vi "DB - [CMS].[Execute].[ActiveProcess].vi"(0 "connection reference":T3, 2 "Application":string, 3 "String ([RawDataFile] Filestream)":string, 4 "[PlantId],[SystemId]":cluster{"[PlantId]":string, "[SystemId]":string}, 5 "error in (no error)":errorcluster, 6 "DB Connection":T4={"Open"=TRUE, "Close"=TRUE}, 7 "Filestream Position (0/<int>/NULL)":string, 8 "DB - CMS Execute ActiveProcess":T2, 9 "Skip TimeStamps":bool, 10 "[Execute].[ActiveProcess]\n2014-10-14 14:58":T1[](array[typedef]), 12 "<Data>":string[](array[string])) -> (14 "connection reference":T3, 15 "data":string[](array[string]), 17 "String ([RawDataFile] Filestream)":string, 19 "SUMMARY":errorcluster)   [LabVIEW 2013]
uses:
  <vilib>/addons/database/Connection.llb/Conn ObjectReference.ctl
  Controls/DB - OpenClose.ctl
  Controls/DB - CMS Execute Active Process.ctl
  Controls/DB - [Execute].[ActiveProcess] Enum.ctl
  Controls/Global CMS.vi
  Controls/Global SRTRS.vi
  <vilib>/addons/database/Connection.llb/DB Tools Open Connec (String).vi
  <vilib>/addons/database/Connection.llb/Conn Execute.vi
  <vilib>/addons/database/Recordset.llb/Rec Destroy - Connection.vi
  <vilib>/addons/database/Recordset.llb/Rec Fetch Recordset Data (R).vi
  <vilib>/addons/database/NI_Database_API.lvlib
panel:
  out "Filestream":string
  out "Close":errorcluster
  out "SQL Statement":string
  in  "DB.Schema.Table \n(NA)":string
  in  "CMS.Execute.ActiveProcess":string="CMS.Execute.ActiveProcess"
  out "CMS Connection Information":T5={"Connection "="SQL Server 32bit HPEnvy", "Username"="admin", "Password"="admin123"}
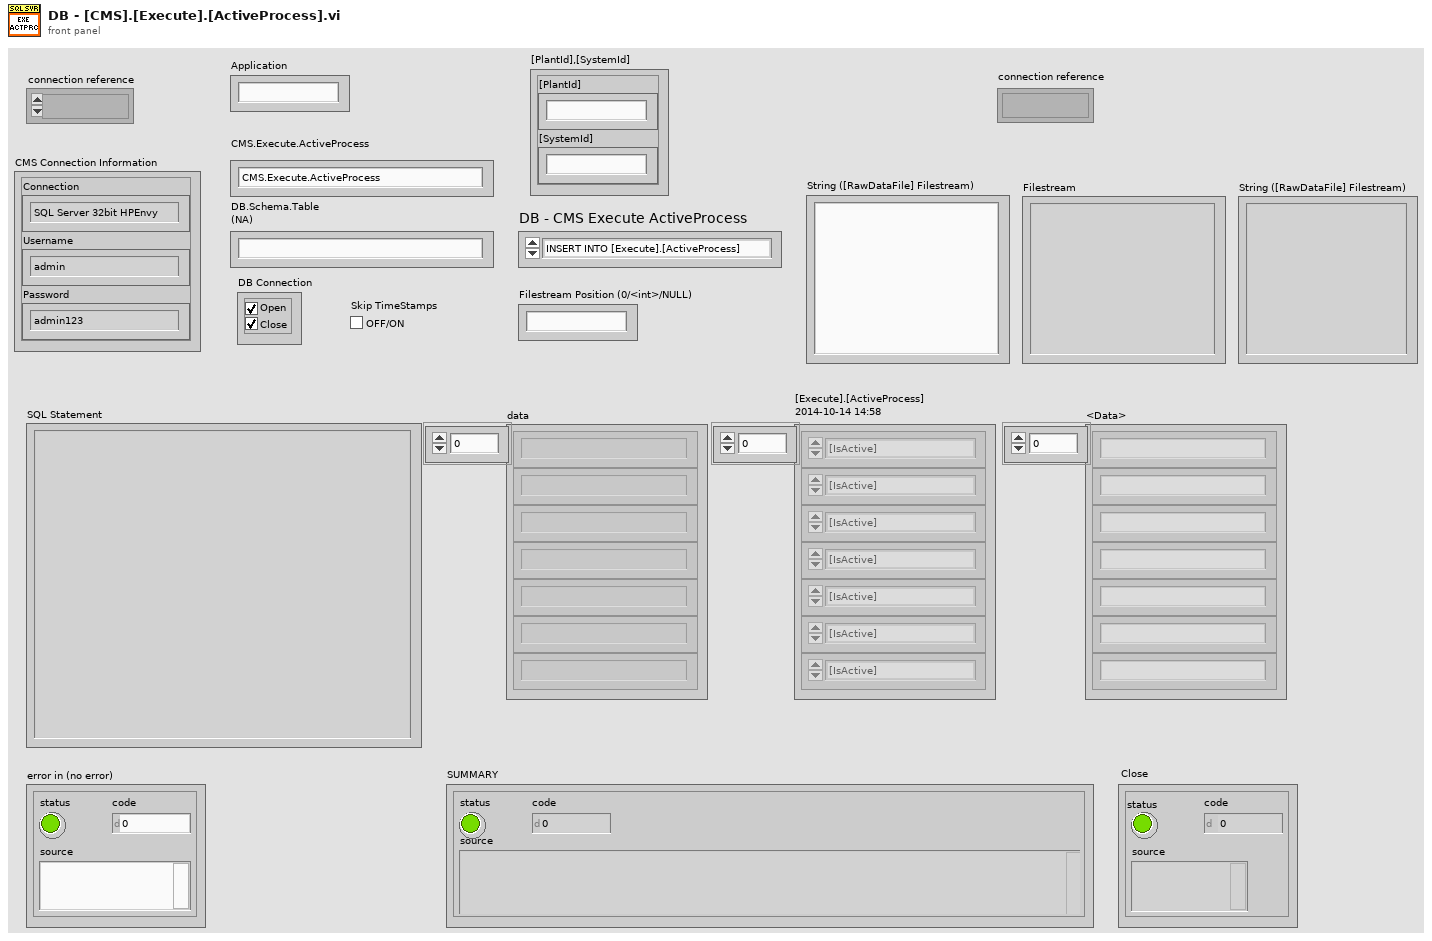
[diagram p1: front panel]
types:
  T1 = typedef "DB - [Execute].[ActiveProcess] Enum.ctl" = enum16{"[IsActive]", "[TransactionNo]", "[TransactionRunNo]", "[SequenceStatus]", "[StartRecordTime]", "[EndRecordTime]", "[StartHoldTime]", "[EndHoldTime]", "[Message1]", "[Message2]", "[HoldTimeRemaining]", "[HoldTimePercentage]", "[HoldProgressColor]", "[OrderNumbers]", "[CurrentTemp]", "[UnitOfTemperature]", "[IsAppClientLive]", "[RawDataFile]", "[RecordedMinutes]", "[FurnaceControlStatus]", "[FurnaceControlColor]", "[ControllerStatus]", "[ControllerColor]", "[IsControllerOnline]", "[ProcessColor]", "[OverallColor]", "[LastUpdatedOn]", "[LastUpdatedCmsTime]", "[Inactive]"}
  T2 = typedef "DB - CMS Execute Active Process.ctl" = enum16{"INSERT INTO [Execute].[ActiveProcess]", "UPDATE [Execute].[ActiveProcess]", "SELECT [Execute].[ActiveProcess]", "UPDATE FILESTREAM", "SELECT FILESTREAM", "Check [IsActive]"}
  T3 = typedef "NI_Database_API.lvlib/Conn ObjectReference.ctl" = refnum<k1>
  T4 = typedef "DB - OpenClose.ctl" = cluster{"Open":bool, "Close":bool}
  T5 = cluster{"Connection ":string, "Username":string, "Password":string}
  T6 = typedef "Enum - InteractiveMode-SubVIMode.ctl" = enum16{"Interactive", "subVI Mode"}
  T7 = typedef "Connection Information Cluster.ctl" = cluster{"Connection ":string, "Username":string, "Password":string}
  T8 = typedef "DB - DB.Schema.Table.ctl" = cluster{"DB":string, "Schema":string, "Table":string}
  T9 = typedef "NI_Database_API.lvlib/Rec ObjectReference.ctl" = refnum<k1>
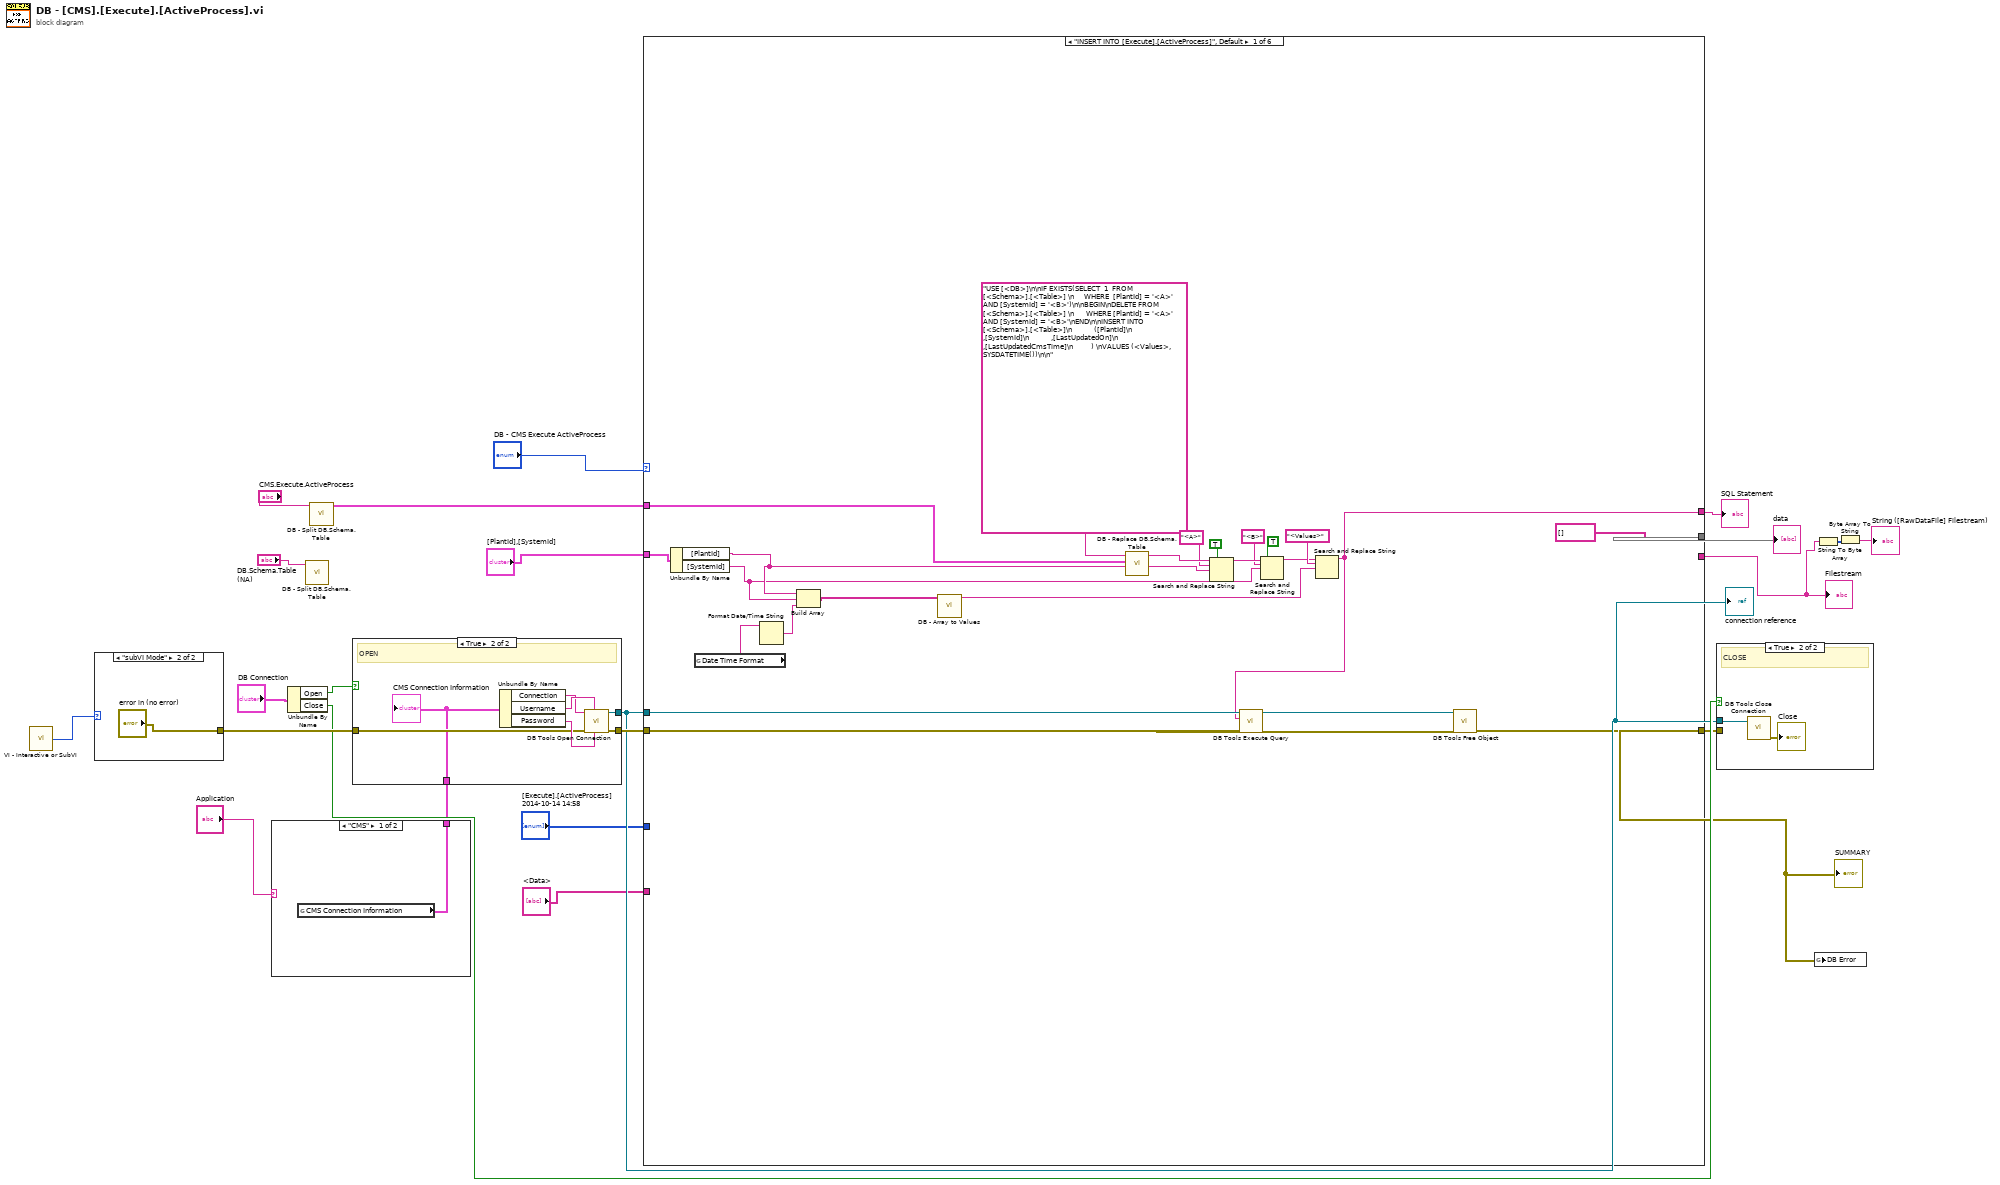
[diagram p0: block diagram]
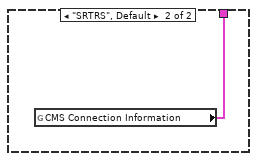
[diagram p2: hidden frame]
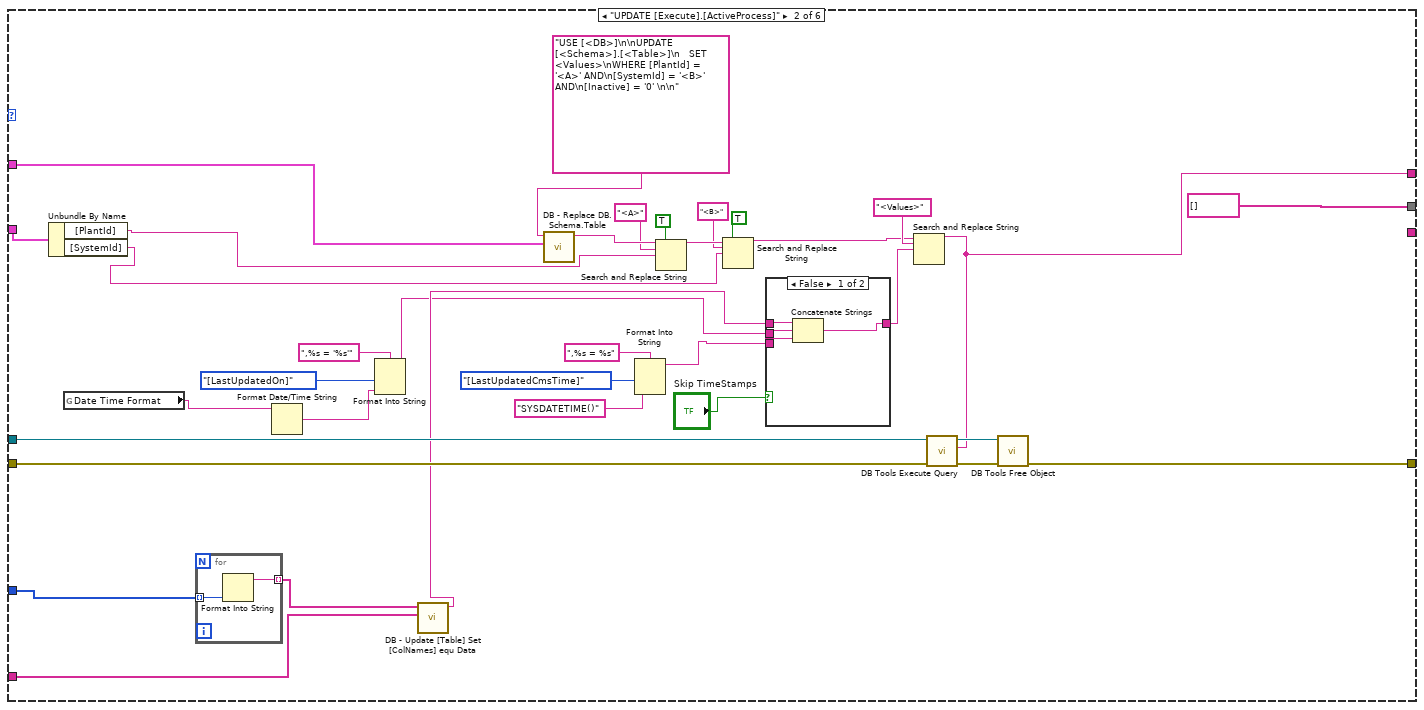
[diagram p3: hidden frame]
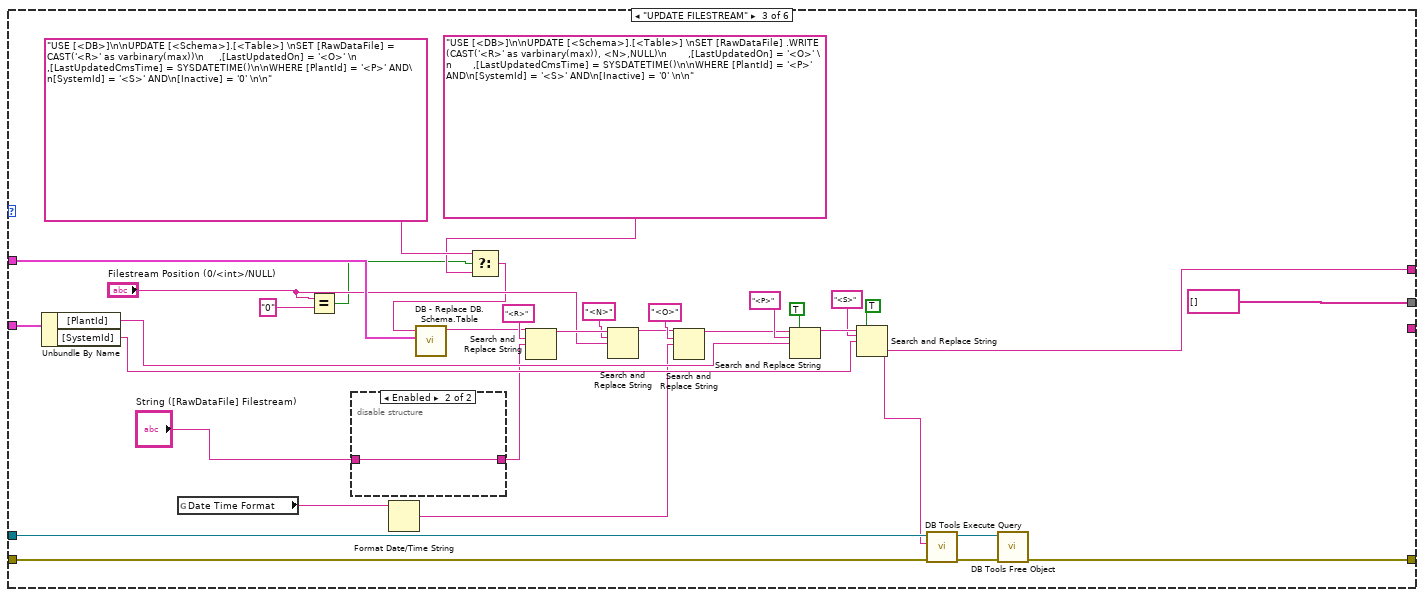
[diagram p5: hidden frame]
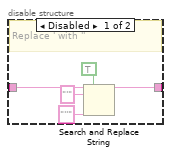
[diagram p6: hidden frame]
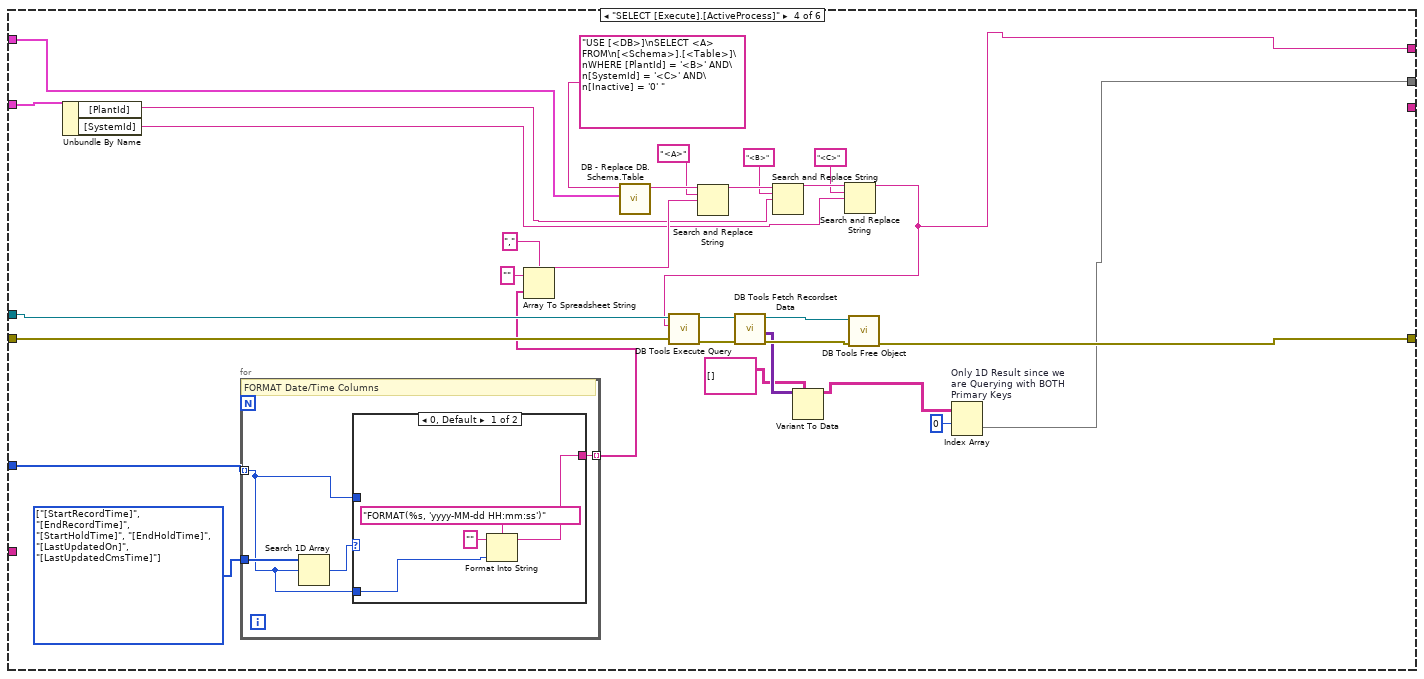
[diagram p7: hidden frame]
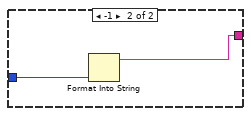
[diagram p8: hidden frame]
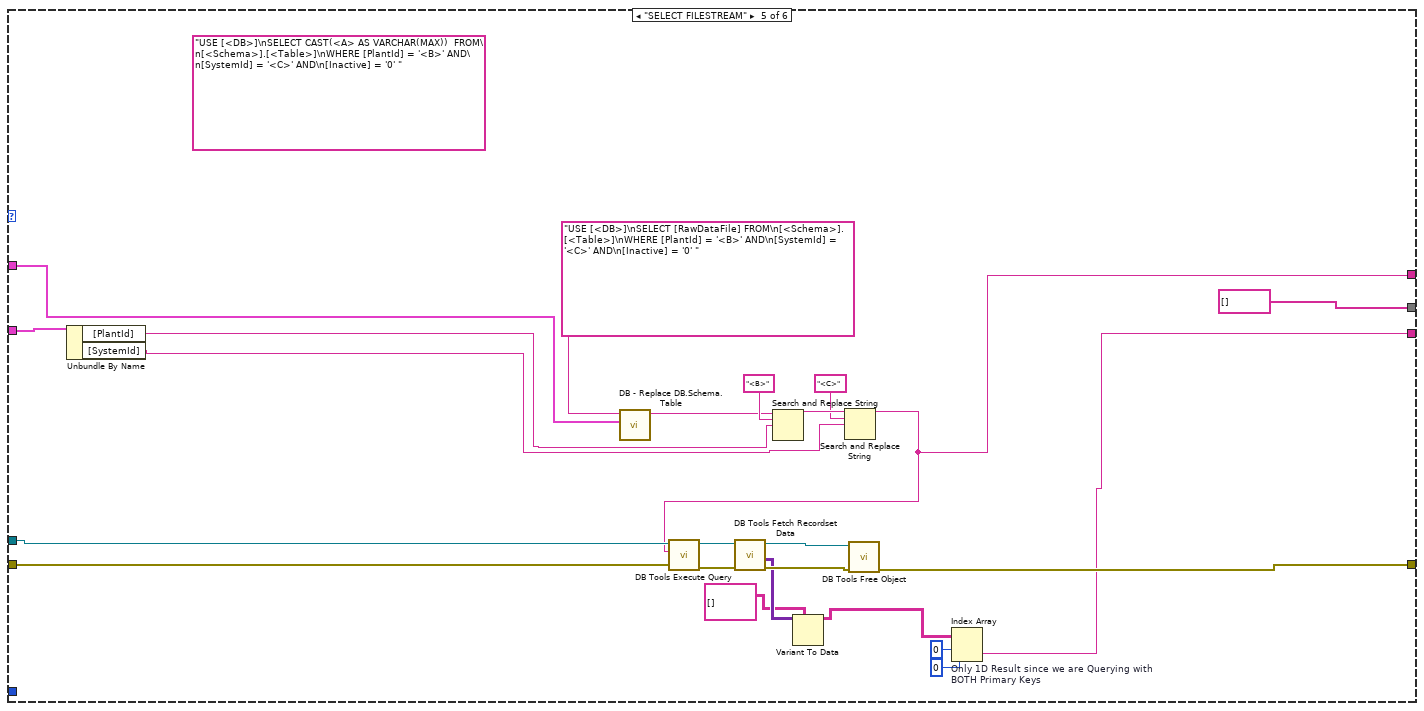
[diagram p9: hidden frame]
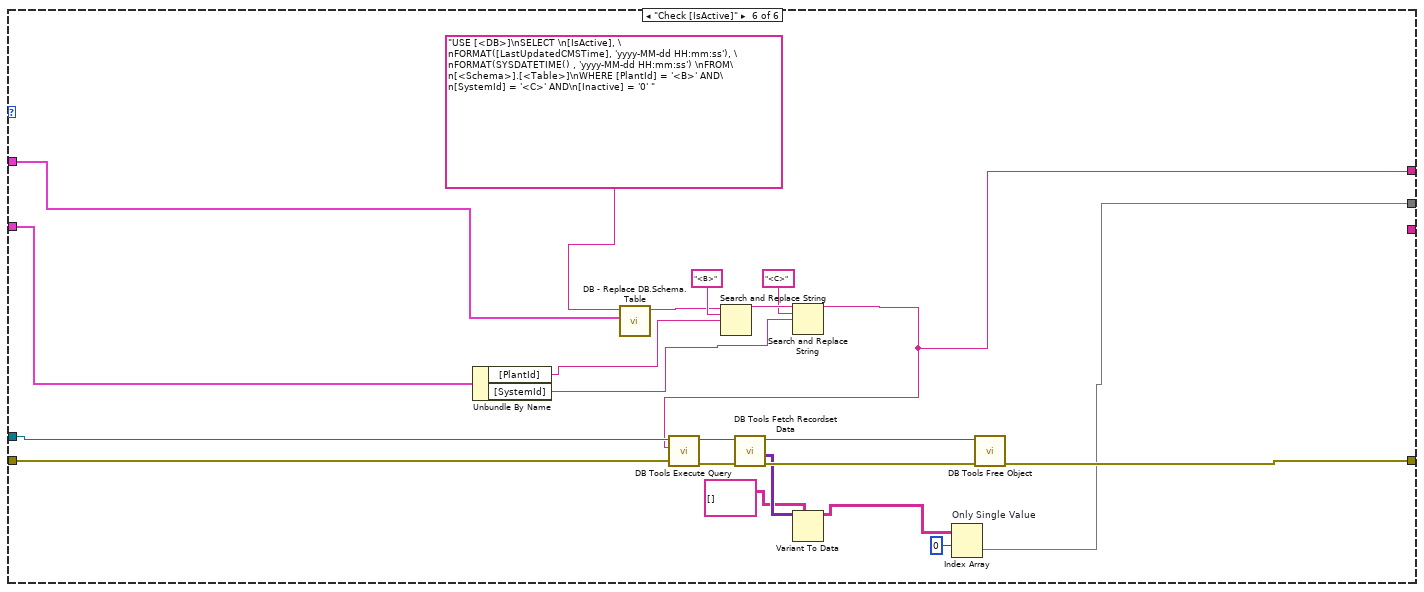
[diagram p10: hidden frame]
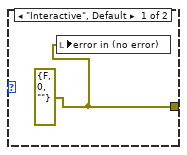
[diagram p12: hidden frame]
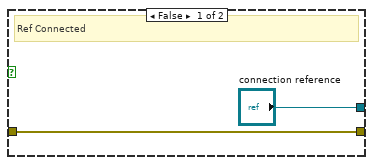
[diagram p13: hidden frame]
diagram:
  n1 = call "VI - Interactive or SubVI.vi"() -> ("Mode"=w20:T6)  [unwired: 5 in]
  n2 = case shown="\"subVI Mode\"" w20 {
    tunnel: [w23 "error in (no error)"] -> w19
    frame "Interactive", Default {
      w23 = errorcluster {"status"=FALSE, "code"=0, "source"=""} ("error in (no error)")
      n3 = local write "error in (no error)"(w23) -> ()
    }
    frame "subVI Mode" {
    }
  }
  n4 = case shown="\"CMS\"" "Application" {
    tunnel: [w25 w26] -> w1
    frame "CMS" {
      n5 = global read "Global CMS.vi" "CMS Connection Information"() -> (w25:T7)
    }
    frame "SRTRS", Default {
      n6 = global read "Global SRTRS.vi" "CMS Connection Information"() -> (w26:T7)
    }
  }
  n7 = Unbundle By Name("DB Connection") -> ("Open"=w21:bool, "Close"=w17:bool)
  n8 = call "DB - Split DB.Schema.Table.vi"("DB.Schema.Table"="DB.Schema.Table \n(NA)") -> ()  [unwired: 10 in, 1 out]
  n9 = call "DB - Split DB.Schema.Table.vi"("DB.Schema.Table"="CMS.Execute.ActiveProcess") -> ("DB.Schema.Table"=w14:T8)  [unwired: 10 in]
  n10 = case shown="True" w21 {
    tunnel: ["connection reference" w32] -> w10
    tunnel: w19 -> [w27 w31]
    tunnel: [w27 w30] -> w18
    tunnel: w1 -> [_ w29]
    frame False {
      # "Ref Connected"
    }
    frame True {
      # "OPEN"
      n11 = Unbundle By Name(w29) -> ("Connection"=w34:string, "Username"=w35:string, "Password"=w33:string)
      n12 = call-poly <vilib>:"DB Tools Open Connection.vi"("password"=w33, "userID"=w35, "error in (no error)"=w31, "connection information"=w34) -> ("error out"=w30:errorcluster, "connection reference"=w32:T3)  [unwired: 4 in]
      "CMS Connection Information" <- w29
    }
  }
  "connection reference" <- w10
  n13 = case shown="\"INSERT INTO [Execute].[ActiveProcess]\", Default" "DB - CMS Execute ActiveProcess" {
    tunnel: w10 -> [w59 w83 w127 w152 w192 w218]
    tunnel: w18 -> [w58 w84 w128 w151 w191 w217]
    tunnel: w14 -> [w57 w86 w129 w147 w188 w215]
    tunnel: [w54 w80 w124 w150 w190 w216] -> w13
    tunnel: [w46 w79 w120 w148 w189 w208] -> w12
    tunnel: "[Execute].[ActiveProcess]\n2014-10-14 14:58" -> [_ w67 _ w143 _ _]
    tunnel: "<Data>" -> [_ w65 _ _ _ _]
    tunnel: [string[] [] string[] [] string[] [] w149 string[] [] w213] -> w7
    tunnel: [_ _ _ _ w185 _] -> w4
    tunnel: "[PlantId],[SystemId]" -> [w38 w74 w119 w146 w184 w207]
    frame "INSERT INTO [Execute].[ActiveProcess]", Default {
      n14 = Unbundle By Name(w38) -> ("[PlantId]"=w37:string, "[SystemId]"=w36:string)
      n15 = global read "Global SRTRS.vi" "Date Time Format"() -> (w40:string)
      n16 = Format Date/Time String(time format string (%c)=w40) -> (date/time string=w39:string)  [unwired: 2 in]
      n17 = Build Array(w37, w36, w39) -> (w41:string[])
      n18 = call "DB - Array to Values.vi"("Array (0xFFFE autodetect)"=w41) -> ("<Values>"=w45:string)  [unwired: 10 in]
      n19 = call "DB - Replace DB.Schema.Table.vi"("DB.Schema.Table"=w57, "string in"="USE [<DB>]\n\nIF EXISTS(SELECT  1  FROM [<Schema>].[<Table>] \n     WHERE  [PlantId] = '<A>'  AND [SystemId] = '<B>')\n\nBEGIN\nDELETE FROM [<Schema>].[<Table>] \n      WHERE [PlantId] = '<A>'  AND [SystemId] = '<B>'\nEND\n\nINSERT INTO [<Schema>].[<Table>]\n           ([PlantId]\n           ,[SystemId]\n           ,[LastUpdatedOn]\n           ,[LastUpdatedCmsTime]\n         ) \nVALUES (<Values>, SYSDATETIME())\n\n") -> ("string out"=w56:string)  [unwired: 8 in, 1 out]
      n20 = Search and Replace String(replace all?=TRUE ("replace all? (F)"), input string=w56, search string="<A>", replace string=w37) -> (result string=w52:string)  [unwired: 4 in, 3 out]
      n21 = Search and Replace String(replace all?=TRUE ("replace all? (F)"), input string=w52, search string="<B>", replace string=w36) -> (result string=w47:string)  [unwired: 4 in, 3 out]
      n22 = Search and Replace String(input string=w47, search string="<Values>", replace string=w45) -> (result string=w46:string)  [unwired: 5 in, 3 out]
      n23 = call-poly <vilib>:"DB Tools Execute Query.vi"("error in (no error)"=w58, "SQL query"=w46, "connection reference"=w59) -> ("error out"=w43:errorcluster, "recordset reference"=w44:T9)  [unwired: 5 in]
      n24 = call-poly <vilib>:"DB Tools Free Object.vi"("error in (no error)"=w43, "recordset reference"=w44) -> ("error out"=w54:errorcluster)  [unwired: 8 in, 1 out]
    }
    frame "UPDATE [Execute].[ActiveProcess]" {
      n25 = Unbundle By Name(w74) -> ("[PlantId]"=w73:string, "[SystemId]"=w72:string)
      n26 = global read "Global SRTRS.vi" "Date Time Format"() -> (w68:string)
      n27 = for {
        tunnel: w67 -> [w101] mode=indexing
        tunnel: [w100] -> w66 mode=indexing
        n28 = Format Into String(w101) -> (resulting string=w100:string)  [unwired: 3 in, 1 out]
      }
      n29 = Format Date/Time String(time format string (%c)=w68) -> (date/time string=w69:string)  [unwired: 2 in]
      n30 = Format Into String(format string=",%s = '%s'", DB_-_[Execute].[ActiveProcess]_Enum."[LastUpdatedOn]" ("[Execute].[ActiveProcess]\n2014-10-14 14:58"), w69) -> (resulting string=w62:string)  [unwired: 2 in, 1 out]
      n31 = call "DB - Update [Table] Set [ColNames] equ Data.vi"("<Data> (0xFFFE autodetect)"=w65, "[ColumnNames]"=w66) -> ("<Values>"=w64:string)  [unwired: 9 in]
      n32 = call "DB - Replace DB.Schema.Table.vi"("DB.Schema.Table"=w86, "string in"="USE [<DB>]\n\nUPDATE [<Schema>].[<Table>]\n   SET <Values>\nWHERE [PlantId] = '<A>' AND\n[SystemId] = '<B>' AND\n[Inactive] = '0' \n\n") -> ("string out"=w94:string)  [unwired: 8 in, 1 out]
      n33 = Format Into String(format string=",%s = %s", DB_-_[Execute].[ActiveProcess]_Enum."[LastUpdatedCmsTime]" ("[Execute].[ActiveProcess]\n2014-10-14 14:58"), "SYSDATETIME()") -> (resulting string=w61:string)  [unwired: 2 in, 1 out]
      n34 = Search and Replace String(replace all?=TRUE ("replace all? (F)"), input string=w94, search string="<A>", replace string=w73) -> (result string=w92:string)  [unwired: 4 in, 3 out]
      n35 = Search and Replace String(replace all?=TRUE ("replace all? (F)"), input string=w92, search string="<B>", replace string=w72) -> (result string=w87:string)  [unwired: 4 in, 3 out]
      n36 = case shown="False" "Skip TimeStamps" {
        tunnel: w64 -> [w98 w99]
        tunnel: [w97 w99] -> w63
        tunnel: w62 -> [w96 _]
        tunnel: w61 -> [w95 _]
        frame False {
          n37 = Concatenate Strings(w98, w96, w95) -> (w97:string)
        }
        frame True {
        }
      }
      n38 = Search and Replace String(input string=w87, search string="<Values>", replace string=w63) -> (result string=w79:string)  [unwired: 5 in, 3 out]
      n39 = call-poly <vilib>:"DB Tools Execute Query.vi"("error in (no error)"=w84, "SQL query"=w79, "connection reference"=w83) -> ("error out"=w82:errorcluster, "recordset reference"=w81:T9)  [unwired: 5 in]
      n40 = call-poly <vilib>:"DB Tools Free Object.vi"("error in (no error)"=w82, "recordset reference"=w81) -> ("error out"=w80:errorcluster)  [unwired: 8 in, 1 out]
    }
    frame "UPDATE FILESTREAM" {
      n41 = Unbundle By Name(w119) -> ("[PlantId]"=w118:string, "[SystemId]"=w117:string)
      n42 = global read "Global SRTRS.vi" "Date Time Format"() -> (w103:string)
      n43 = Equal?(x="Filestream Position (0/<int>/NULL)", y="0") -> (x = y?=w107:bool)
      n44 = disable-structure shown="Enabled" {
        disable-tunnel: "String ([RawDataFile] Filestream)" -> [w139 w140]
        disable-tunnel: [w138 w140] -> w115
        frame Disabled {
          # "Replace ' with ''"
          n45 = Search and Replace String(replace all?=TRUE ("replace all? (F)"), input string=w139, search string="'", replace string="''" ("replace string (\"\")")) -> (result string=w138:string)  [unwired: 4 in, 3 out]
        }
        frame Enabled {
        }
      }
      n46 = Format Date/Time String(time format string (%c)=w103) -> (date/time string=w102:string)  [unwired: 2 in]
      n47 = Select(t="USE [<DB>]\n\nUPDATE [<Schema>].[<Table>] \nSET [RawDataFile] = CAST('<R>' as varbinary(max))\n     ,[LastUpdatedOn] = '<O>' \n     ,[LastUpdatedCmsTime] = SYSDATETIME()\n\nWHERE [PlantId] = '<P>' AND\n[SystemId] = '<S>' AND\n[Inactive] = '0' \n\n", s=w107, f="USE [<DB>]\n\nUPDATE [<Schema>].[<Table>] \nSET [RawDataFile] .WRITE (CAST('<R>' as varbinary(max)), <N>,NULL)\n       ,[LastUpdatedOn] = '<O>' \n       ,[LastUpdatedCmsTime] = SYSDATETIME()\n\nWHERE [PlantId] = '<P>' AND\n[SystemId] = '<S>' AND\n[Inactive] = '0' \n\n") -> (s? t:f=w108:string)
      n48 = call "DB - Replace DB.Schema.Table.vi"("DB.Schema.Table"=w129, "string in"=w108) -> ("string out"=w121:string)  [unwired: 8 in, 1 out]
      n49 = Search and Replace String(input string=w121, search string="<R>", replace string=w115) -> (result string=w114:string)  [unwired: 5 in, 3 out]
      n50 = Search and Replace String(input string=w114, search string="<N>", replace string="Filestream Position (0/<int>/NULL)") -> (result string=w104:string)  [unwired: 5 in, 3 out]
      n51 = Search and Replace String(input string=w104, search string="<O>", replace string=w102) -> (result string=w105:string)  [unwired: 5 in, 3 out]
      n52 = Search and Replace String(replace all?=TRUE ("replace all? (F)"), input string=w105, search string="<P>", replace string=w118) -> (result string=w133:string)  [unwired: 4 in, 3 out]
      n53 = Search and Replace String(replace all?=TRUE ("replace all? (F)"), input string=w133, search string="<S>", replace string=w117) -> (result string=w120:string)  [unwired: 4 in, 3 out]
      n54 = call-poly <vilib>:"DB Tools Execute Query.vi"("error in (no error)"=w128, "SQL query"=w120, "connection reference"=w127) -> ("error out"=w126:errorcluster, "recordset reference"=w125:T9)  [unwired: 5 in]
      n55 = call-poly <vilib>:"DB Tools Free Object.vi"("error in (no error)"=w126, "recordset reference"=w125) -> ("error out"=w124:errorcluster)  [unwired: 8 in, 1 out]
    }
    frame "SELECT [Execute].[ActiveProcess]" {
      w142 = T1[] [enum."[StartRecordTime]", enum."[EndRecordTime]", enum."[StartHoldTime]", enum."[EndHoldTime]", enum."[LastUpdatedOn]", enum."[LastUpdatedCmsTime]"] items=["[IsActive]", "[TransactionNo]", "[TransactionRunNo]", "[SequenceStatus]", "[StartRecordTime]", "[EndRecordTime]", "[StartHoldTime]", "[EndHoldTime]", "[Message1]", "[Message2]", "[HoldTimeRemaining]", "[HoldTimePercentage]", "[HoldProgressColor]", "[OrderNumbers]", "[CurrentTemp]", "[UnitOfTemperature]", "[IsAppClientLive]", "[RawDataFile]", "[RecordedMinutes]", "[FurnaceControlStatus]", "[FurnaceControlColor]", "[ControllerStatus]", "[ControllerColor]", "[IsControllerOnline]", "[ProcessColor]", "[OverallColor]", "[LastUpdatedOn]", "[LastUpdatedCmsTime]", "[Inactive]"] ("[Execute].[ActiveProcess]\n2014-10-14 14:58")
      n56 = Unbundle By Name(w146) -> ("[PlantId]"=w145:string, "[SystemId]"=w144:string)
      n57 = for {
        tunnel: w143 -> [w171] mode=indexing
        tunnel: [w172] -> w141 mode=indexing
        tunnel: w142 -> [w174]
        # "FORMAT Date/Time Columns"
        n58 = Search 1D Array(1D array=w174, element=w171) -> (index of element=w173:i32)  [unwired: 1 in]
        n59 = case shown="0, Default" w173 {
          tunnel: w171 -> [w176 _]
          tunnel: [w175 w179] -> w172
          tunnel: w171 -> [_ w180]
          frame 0, Default {
            n60 = Format Into String(format string="FORMAT(%s, 'yyyy-MM-dd HH:mm:ss')", initial string="", w176) -> (resulting string=w175:string)  [unwired: 1 in, 1 out]
          }
          frame -1 {
            n61 = Format Into String(w180) -> (resulting string=w179:string)  [unwired: 3 in, 1 out]
          }
        }
      }
      n62 = Array To Spreadsheet String(delimiter (Tab)=",", array=w141, 3:"" ("format string")) -> (spreadsheet string=w157:string)
      n63 = call "DB - Replace DB.Schema.Table.vi"("DB.Schema.Table"=w147, "string in"="USE [<DB>]\nSELECT <A> FROM\n[<Schema>].[<Table>]\nWHERE [PlantId] = '<B>' AND\n[SystemId] = '<C>' AND\n[Inactive] = '0' ") -> ("string out"=w169:string)  [unwired: 8 in, 1 out]
      n64 = Search and Replace String(input string=w169, search string="<A>", replace string=w157) -> (result string=w167:string)  [unwired: 5 in, 3 out]
      n65 = Search and Replace String(input string=w167, search string="<B>", replace string=w145) -> (result string=w165:string)  [unwired: 5 in, 3 out]
      n66 = Search and Replace String(input string=w165, search string="<C>", replace string=w144) -> (result string=w148:string)  [unwired: 5 in, 3 out]
      n67 = call-poly <vilib>:"DB Tools Execute Query.vi"("error in (no error)"=w151, "SQL query"=w148, "connection reference"=w152) -> ("error out"=w161:errorcluster, "recordset reference"=w163:T9)  [unwired: 5 in]
      n68 = call-poly <vilib>:"DB Tools Fetch Recordset Data.vi"("error in (no error)"=w161, "recordset reference"=w163) -> ("error out"=w160:errorcluster, "recordset data"=w159:variant[][], "recordset reference out"=w162:T9)  [unwired: 3 in]
      n69 = Variant To Data(type=string[][] [], Variant=w159) -> (data=w154:string[][])  [unwired: 1 in, 1 out]
      n70 = call-poly <vilib>:"DB Tools Free Object.vi"("error in (no error)"=w160, "recordset reference"=w162) -> ("error out"=w150:errorcluster)  [unwired: 8 in, 1 out]
      n71 = Index Array "Only 1D Result since we are Querying with BOTH Primary Keys"(array=w154, index (row)=0) -> (element=w149:string[])  [unwired: 1 in]
    }
    frame "SELECT FILESTREAM" {
      (unwired) "USE [<DB>]\nSELECT CAST(<A> AS VARCHAR(MAX))  FROM\n[<Schema>].[<Table>]\nWHERE [PlantId] = '<B>' AND\n[SystemId] = '<C>' AND\n[Inactive] = '0' "
      n72 = Unbundle By Name(w184) -> ("[PlantId]"=w183:string, "[SystemId]"=w182:string)
      n73 = call "DB - Replace DB.Schema.Table.vi"("DB.Schema.Table"=w188, "string in"="USE [<DB>]\nSELECT [RawDataFile] FROM\n[<Schema>].[<Table>]\nWHERE [PlantId] = '<B>' AND\n[SystemId] = '<C>' AND\n[Inactive] = '0' ") -> ("string out"=w181:string)  [unwired: 8 in, 1 out]
      n74 = Search and Replace String(input string=w181, search string="<B>", replace string=w183) -> (result string=w202:string)  [unwired: 5 in, 3 out]
      n75 = Search and Replace String(input string=w202, search string="<C>", replace string=w182) -> (result string=w189:string)  [unwired: 5 in, 3 out]
      n76 = call-poly <vilib>:"DB Tools Execute Query.vi"("error in (no error)"=w191, "SQL query"=w189, "connection reference"=w192) -> ("error out"=w198:errorcluster, "recordset reference"=w200:T9)  [unwired: 5 in]
      n77 = call-poly <vilib>:"DB Tools Fetch Recordset Data.vi"("error in (no error)"=w198, "recordset reference"=w200) -> ("error out"=w197:errorcluster, "recordset data"=w196:variant[][], "recordset reference out"=w199:T9)  [unwired: 3 in]
      n78 = Variant To Data(type=string[][] [], Variant=w196) -> (data=w194:string[][])  [unwired: 1 in, 1 out]
      n79 = call-poly <vilib>:"DB Tools Free Object.vi"("error in (no error)"=w197, "recordset reference"=w199) -> ("error out"=w190:errorcluster)  [unwired: 8 in, 1 out]
      n80 = Index Array "Only 1D Result since we are Querying with BOTH Primary Keys"(array=w194, index (row)=0, index (col)=0 ("disabled index (col)")) -> (element=w185:string)
    }
    frame "Check [IsActive]" {
      n81 = Unbundle By Name(w207) -> ("[PlantId]"=w206:string, "[SystemId]"=w205:string)
      n82 = call "DB - Replace DB.Schema.Table.vi"("DB.Schema.Table"=w215, "string in"="USE [<DB>]\nSELECT \n[IsActive], \nFORMAT([LastUpdatedCMSTime], 'yyyy-MM-dd HH:mm:ss'), \nFORMAT(SYSDATETIME() , 'yyyy-MM-dd HH:mm:ss') \nFROM\n[<Schema>].[<Table>]\nWHERE [PlantId] = '<B>' AND\n[SystemId] = '<C>' AND\n[Inactive] = '0' ") -> ("string out"=w209:string)  [unwired: 8 in, 1 out]
      n83 = Search and Replace String(input string=w209, search string="<B>", replace string=w206) -> (result string=w211:string)  [unwired: 5 in, 3 out]
      n84 = Search and Replace String(input string=w211, search string="<C>", replace string=w205) -> (result string=w208:string)  [unwired: 5 in, 3 out]
      n85 = call-poly <vilib>:"DB Tools Execute Query.vi"("error in (no error)"=w217, "SQL query"=w208, "connection reference"=w218) -> ("error out"=w224:errorcluster, "recordset reference"=w226:T9)  [unwired: 5 in]
      n86 = call-poly <vilib>:"DB Tools Fetch Recordset Data.vi"("error in (no error)"=w224, "recordset reference"=w226) -> ("error out"=w223:errorcluster, "recordset data"=w222:variant[][], "recordset reference out"=w225:T9)  [unwired: 3 in]
      n87 = Variant To Data(type=string[][] [], Variant=w222) -> (data=w220:string[][])  [unwired: 1 in, 1 out]
      n88 = Index Array "Only Single Value"(array=w220, index (row)=0) -> (element=w213:string[])  [unwired: 1 in]
      n89 = call-poly <vilib>:"DB Tools Free Object.vi"("error in (no error)"=w223, "recordset reference"=w225) -> ("error out"=w216:errorcluster)  [unwired: 8 in, 1 out]
    }
  }
  "SUMMARY" <- w13
  "SQL Statement" <- w12
  "data" <- w7
  "Filestream" <- w4
  n90 = case shown="True" w17 {
    tunnel: w10 -> [_ w228]
    tunnel: w13 -> [_ _]
    frame False {
      # "Ref Connected"
    }
    frame True {
      # "CLOSE"
      n91 = call <vilib>:"DB Tools Close Connection.vi"("connection reference"=w228) -> ("error out"=→"Close":errorcluster)  [unwired: 6 in]
    }
  }
  n92 = global write "Global SRTRS.vi" "DB Error"(w13) -> ()
  n93 = String To Byte Array(string=w4) -> (unsigned byte array=w6:u8[])
  n94 = Byte Array To String(unsigned byte array=w6) -> (string=→"String ([RawDataFile] Filestream)":string)
